vi "CAM TEST.vi"() -> ()   [LabVIEW 2020]
uses:
  F:/MY FILE/FaceRecognitionDotNet 1.2.3.10/FaceRecognitionDotNet/FaceRecognition Class/dll/FaceRecognitionDotNet.dll
  FaceRecognitionDotNet/FaceRecognition Class/dll/FaceRecognitionDotNet.dll
  FaceRecognitionDotNet/FaceRecognition Class/ctl/LocationModel.ctl
  FaceRecognitionDotNet/FaceRecognition Class/FaceRecognition.lvclass
  <vilib>/vision/driver/NI_Vision_Acquisition_Software.lvlib
  <vilib>/vision/NI_Vision_Development_Module.lvlib
panel:
  in  "Landmark path":path=path "C:/Users/foxlink/Desktop/builds/netstandard2.0/img/003.bin"
  in  "mode path":path=path "C:/Users/foxlink/Desktop/builds/netstandard2.0/Class/models"
  out "element":dbl
  out "Processed Frames/s":dbl
  out "Acquired Frames/s":dbl
  in  "Cancel Button":bool
  out "Image":T1(plugin-control)
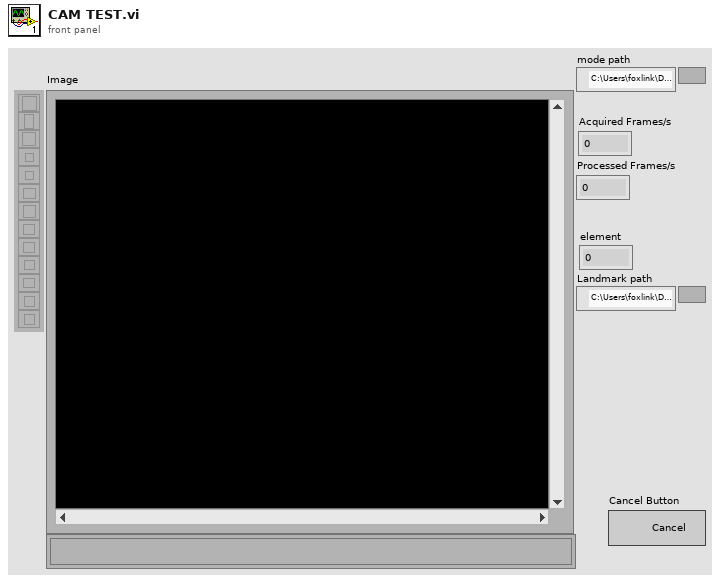
[diagram p1: front panel]
types:
  T1 = typedef "IMAQ Image.ctl" = refnum<image>
  T2 = typedef "Image Type" = u32
  T3 = cluster{"Type":u32, "Version":u32, "Flags":u32, "SerialNumberHigh":u32, "SerialNumberLow":u32, "BusType":u32, "InterfaceName":string, "VendorName":string, "ModelName":string, "CameraFileName":string, "CameraAttributeURL":string}[]
  T4 = cluster{"Type":u32, "Version":u32, "Flags":u32, "SerialNumberHigh":u32, "SerialNumberLow":u32, "BusType":u32, "InterfaceName":string, "VendorName":string, "ModelName":string, "CameraFileName":string, "CameraAttributeURL":string}
  T5 = typedef "IMAQdx.ctl" = refnum<k21>
  T6 = typedef "FaceRecognitionDotNet.lvlib/FaceRecognition.lvclass/LocationModel.ctl" = i32
  T7 = cluster{"DataArray":u8[], "rows":i32, "columns":i32, "elementSize":i32}
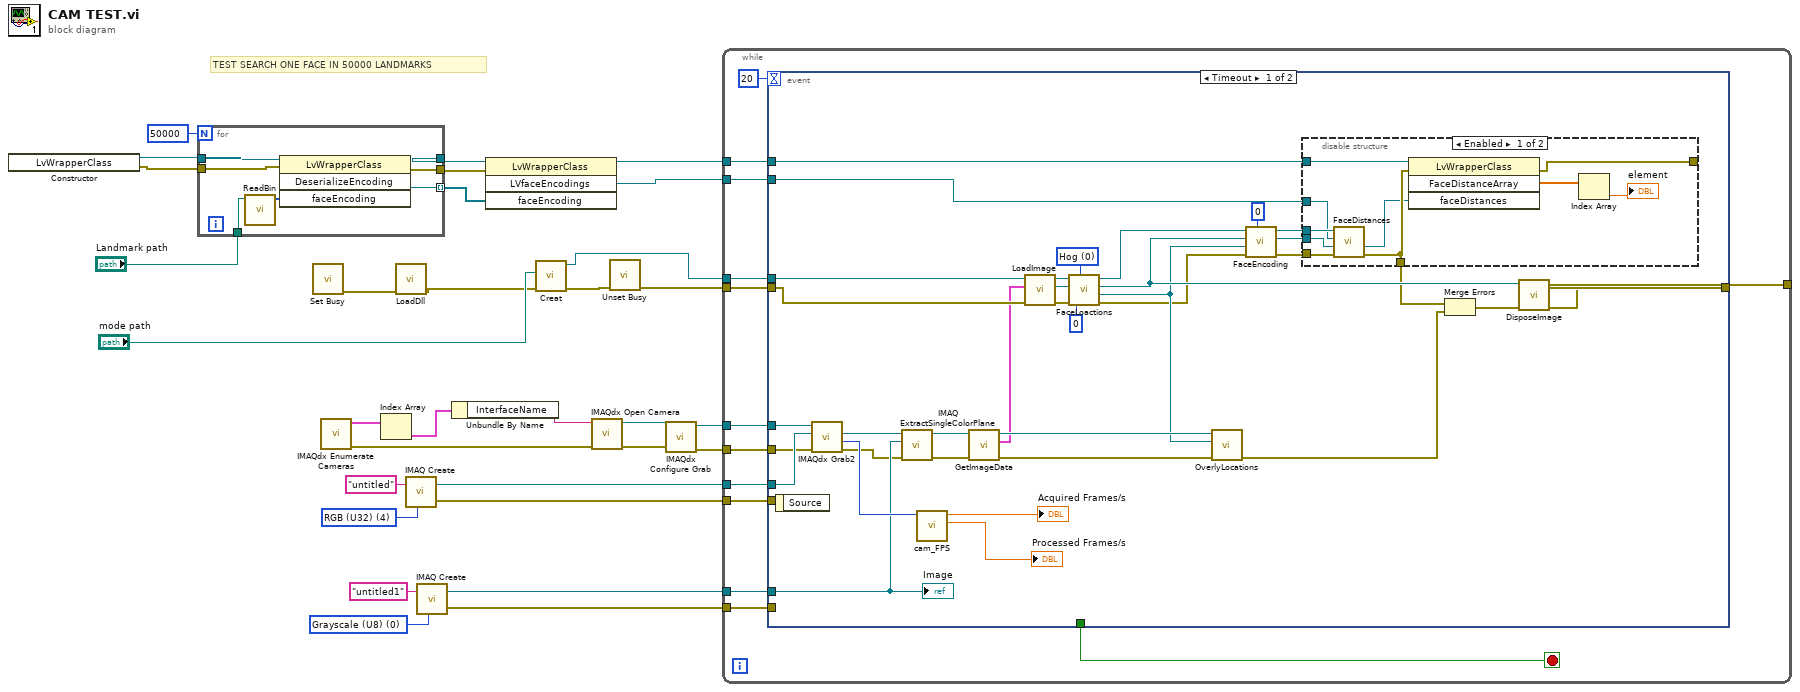
[diagram p0: block diagram]
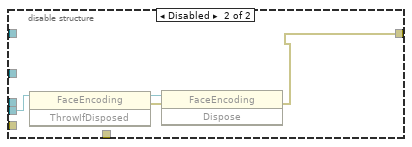
[diagram p2: hidden frame]
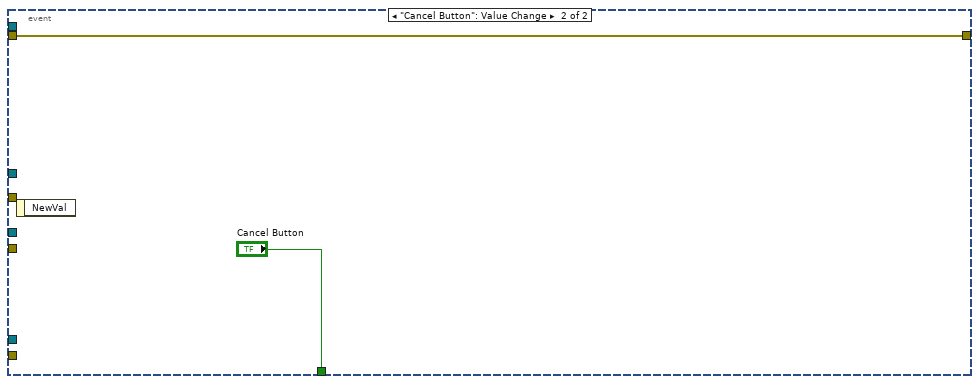
[diagram p3: hidden frame]
diagram:
  w7 = T2 0 items=["Grayscale (U8)", "Grayscale (I16)", "Grayscale (SGL)", "Complex (CSG)", "RGB (U32)", "HSL (U32)", "RGB (U64)", "Grayscale (U16)"] ("Image Type")
  w28 = T2 4 items=["Grayscale (U8)", "Grayscale (I16)", "Grayscale (SGL)", "Complex (CSG)", "RGB (U32)", "HSL (U32)", "RGB (U64)", "Grayscale (U16)"] ("Image Type")
  # "TEST SEARCH ONE FACE IN 50000 LANDMARKS"
  n1 = constructor class="LvWrapperClass"() -> (reference out=w13:refnum<k24>, error out=w3:errorcluster)  [unwired: 3 in, 1 out]
  n2 = for {
    N: 50000 -> [_]
    tunnel: [w35] -> w14 mode=indexing
    tunnel: w13 -> [w38]
    tunnel: "Landmark path" -> [w36]
    tunnel: w3 -> [w34]
    tunnel: [w33] -> w2
    tunnel: [w32] -> w1
    n3 = call "ReadBin.vi"("FaceEncoding file"=w36) -> ("Array"=w37:u8[])  [unwired: 9 in, 1 out]
    n4 = invoke class="LvWrapperClass" method="DeserializeEncoding"(reference=w38, error in=w34, "faceEncoding"=w37) -> (reference out=w32:refnum<k24>, error out=w33:errorcluster, "DeserializeEncoding"=w35:refnum<k24>)  [unwired: 1 in, 1 out]
  }
  n5 = call <vilib>:"Set Busy.vi"() -> ("error out"=w24:errorcluster)  [unwired: 10 in, 1 out]
  n6 = call <vilib>:"IMAQdx Enumerate Cameras.vi"() -> ("error out"=w18:errorcluster, "Camera Information Array"=w21:T3)  [unwired: 10 in]
  n7 = Index Array(array=w21) -> (element=w20:T4)  [unwired: 1 in]
  n8 = call "LoadDll.vi"("error in (no error)"=w24) -> ("error out"=w23:errorcluster)  [unwired: 10 in]
  n9 = call "IMAQ Create"("Image Name"="untitled", "Image Type"=w28) -> ("New Image"=w31:T1, "error out"=w30:errorcluster)  [unwired: 3 in]
  n10 = call "IMAQ Create"("Image Name"="untitled1", "Image Type"=w7) -> ("New Image"=w5:T1, "error out"=w4:errorcluster)  [unwired: 3 in]
  n11 = Unbundle By Name(w20) -> ("InterfaceName"=w19:string)
  n12 = invoke class="LvWrapperClass" method="LVfaceEncodings"(reference=w1, error in=w2, "faceEncoding"=w14) -> (reference out=w12:refnum<k24>, "LVfaceEncodings"=w11:refnum<k24>)  [unwired: 1 in, 2 out]
  n13 = call "Creat.vi"("error in (no error)"=w23, "mode path"="mode path") -> ("error out"=w26:errorcluster, "FaceRecognition out"=w27:refnum<class "FaceRecognition.lvclass">)  [unwired: 8 in]
  n14 = call <vilib>:"IMAQdx Open Camera.vi"("error in"=w18, "Session In"=w19) -> ("error out"=w17:errorcluster, "Session Out"=w8:T5)  [unwired: 8 in]
  n15 = call <vilib>:"Unset Busy.vi"("error in (no error)"=w26) -> ("error out"=w22:errorcluster)  [unwired: 10 in]
  n16 = call <vilib>:"IMAQdx Configure Grab.vi"("error in"=w17, "Session In"=w8) -> ("error out"=w15:errorcluster, "Session Out"=w16:T5)  [unwired: 8 in]
  n17 = while {
    tunnel: w27 -> [w50]
    tunnel: w22 -> [w49]
    tunnel: w31 -> [w47]
    tunnel: w30 -> [w48]
    tunnel: [w46] -> _
    tunnel: w12 -> [w44]
    tunnel: w16 -> [w43]
    tunnel: w15 -> [w42]
    tunnel: w11 -> [w41]
    tunnel: w5 -> [w40]
    tunnel: w4 -> [w39]
    stop <- w51 stop-if-true
    n18 = event shown="[0] Timeout" {
      selector: _ -> [_ _]
      dyn-events: _ -> [_ _]
      timeout: 20 -> [_ _]
      tunnel: [_ "Cancel Button"] -> w51
      tunnel: w50 -> [w83 _]
      tunnel: w49 -> [w67 w101]
      tunnel: w47 -> [w85 _]
      tunnel: w48 -> [_ _]
      tunnel: [w75 w101] -> w46
      tunnel: w44 -> [w78 _]
      tunnel: w43 -> [w86 _]
      tunnel: w42 -> [w84 _]
      tunnel: w41 -> [w77 _]
      tunnel: w40 -> [w70 _]
      tunnel: w39 -> [_ _]
      event Timeout {
        w59 = T6 0 items=["Hog", "Cnn"] ("model")
        n19 = event-data() -> ()  [unwired: 1 in, 1 out]
        n20 = call <vilib>:"IMAQdx Grab2.vi"("error in"=w84, "Image In"=w85, "Session In"=w86) -> ("error out"=w68:errorcluster, "Buffer Number Out"=w74:u32, "Image Out"=w71:T1)  [unwired: 5 in, 1 out]
        n21 = call "IMAQ ExtractSingleColorPlane"("error in (no error)"=w68, "Image Dst"=w70, "Image Src"=w71) -> ("error out"=w63:errorcluster, "Image Dst Out"=w64:T1)  [unwired: 7 in]
        n22 = call "cam_FPS.vi"("Buffer Number"=w74) -> ("Processed Frames/s"=→"Processed Frames/s":dbl, "Acquired Frames/s"=→"Acquired Frames/s":dbl)  [unwired: 8 in, 1 out]
        n23 = call "GetImageData.vi"("error in (no error)"=w63, "Image"=w64) -> ("error out"=w82:errorcluster, "ImageData Out"=w65:T7, "Image out"=w81:T1)  [unwired: 7 in]
        n24 = call "LoadImage.vi"("error in (no error)"=w67, "ImageData"=w65, "FaceRecognition in"=w83) -> ("error out"=w62:errorcluster, "LoadImage"=w61:refnum<k24>, "FaceRecognition out"=w60:refnum<class "FaceRecognition.lvclass">)  [unwired: 6 in]
        n25 = call "FaceLoactions.vi"("model"=w59, "error in (no error)"=w62, "numberOfTimesToUpsample"=0, "image"=w61, "FaceRecognition in"=w60) -> ("error out"=w69:errorcluster, "FaceLocations"=w76:refnum<k24>, "image out"=w80:refnum<k24>, "FaceRecognition out"=w79:refnum<class "FaceRecognition.lvclass">)  [unwired: 3 in]
        n26 = call "OverlyLocations.vi"("error in (no error)"=w82, "FaceLocations"=w76, "Image in"=w81) -> ("error out"=w57:errorcluster)  [unwired: 6 in, 2 out]
        n27 = call "FaceEncoding.vi"("numJitters"=0, "error in (no error)"=w69, "knownFaceLocation"=w76, "image"=w80, "FaceRecognition in"=w79) -> ("error out"=w54:errorcluster, "FirstFaceEncoding"=w52:refnum<k24>, "FaceRecognition out"=w55:refnum<class "FaceRecognition.lvclass">)  [unwired: 4 in]
        n28 = disable-structure shown="Enabled" {
          disable-tunnel: w55 -> [w96 _]
          disable-tunnel: w54 -> [w95 _]
          disable-tunnel: w77 -> [w94 _]
          disable-tunnel: w52 -> [w93 w100]
          disable-tunnel: w78 -> [w92 _]
          disable-tunnel: [w91 _] -> w66
          disable-tunnel: [w87 w97] -> _
          frame Enabled {
            n29 = call "FaceDistances.vi"("error in (no error)"=w95, "faceToCompare"=w93, "faceEncodings"=w94, "FaceRecognition in"=w96) -> ("error out"=w91:errorcluster, "FaceDistances"=w90:refnum<k24>)  [unwired: 5 in, 1 out]
            n30 = invoke class="LvWrapperClass" method="FaceDistanceArray"(reference=w92, error in=w91, "faceDistances"=w90) -> (error out=w87:errorcluster, "FaceDistanceArray"=w89:dbl[])  [unwired: 1 in, 2 out]
            n31 = Index Array(array=w89) -> (element=→"element":dbl)  [unwired: 1 in]
          }
          frame Disabled {
            n32 = invoke class="FaceEncoding" method="ThrowIfDisposed"(reference=w100) -> (reference out=w99:refnum<k24>, error out=w98:errorcluster)  [unwired: 2 in, 1 out]
            n33 = invoke class="FaceEncoding" method="Dispose"(reference=w99, error in=w98) -> (error out=w97:errorcluster)  [unwired: 1 in, 2 out]
          }
        }
        n34 = Merge Errors(w66, w57) -> (w56:errorcluster)
        n35 = call "DisposeImage.vi"("error in (no error)"=w56, "Image in"=w80) -> ("error out"=w75:errorcluster)  [unwired: 9 in]
        "Image" <- w70
      }
      event "Cancel Button": Value Change {
        n36 = event-data() -> ()  [unwired: 1 in, 1 out]
      }
    }
  }
